vi "EZ Temperature.vi"(0 "VISA Resource Name":refnum<visa-resource-name>, 1 "Scan List (empty)":string, 5 "Thermocouple Type (8:Def-Last)":T2(ring)=enum."Default (Last)", 7 "Thermistor Type (3:Def-Last)":T3(ring)=enum."Default (Last)", 9 "RTD Type (2:Default-Last)":enum16{"85", "91", "Default (Last)"}(ring)=enum."Default (Last)", 11 "error in (no error)":errorcluster, 12 "Transducer Type (4:Def-Last)":T1(ring)=enum."Default (Last)") -> (4 "VISA Resource Name Out":refnum<visa-resource-name>, 8 "Output Array":dbl[](array[numeric]) format="%.2f", 15 "error out":errorcluster)   [LabVIEW 2016, in "Agilent 34970.lvlib"]
doc: "This VI lets you take simple temperature measurements. You can use various types of thermocouples, thermistors, or RTDs."
uses:
  Agilent 34970.lvlib
panel:
  out "concatenated string":string
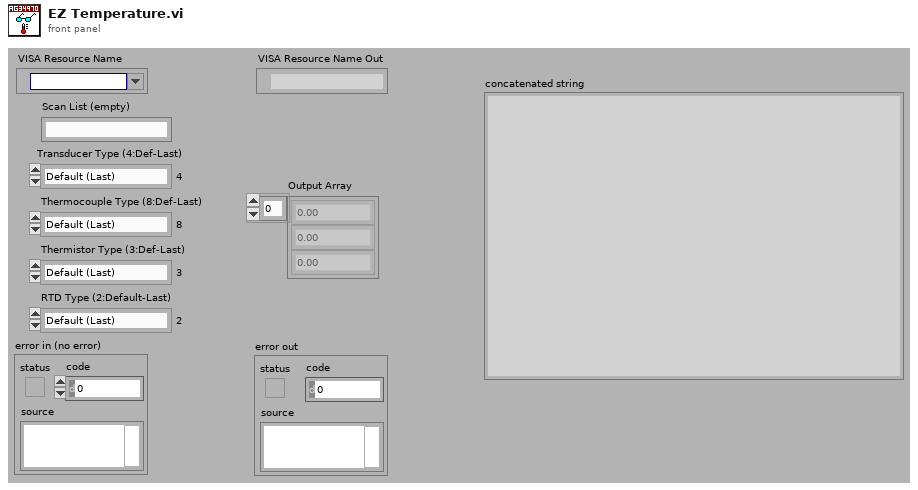
[diagram p1: front panel]
types:
  T1 = enum16{"Thermocouple", "Thermistor", "RTD", "4-Wire RTD", "Default (Last)"}
  T2 = enum16{"B", "E", "J", "K", "N", "R", "S", "T", "Default (Last)"}
  T3 = enum16{"2252", "5000", "10000", "Default (Last)"}
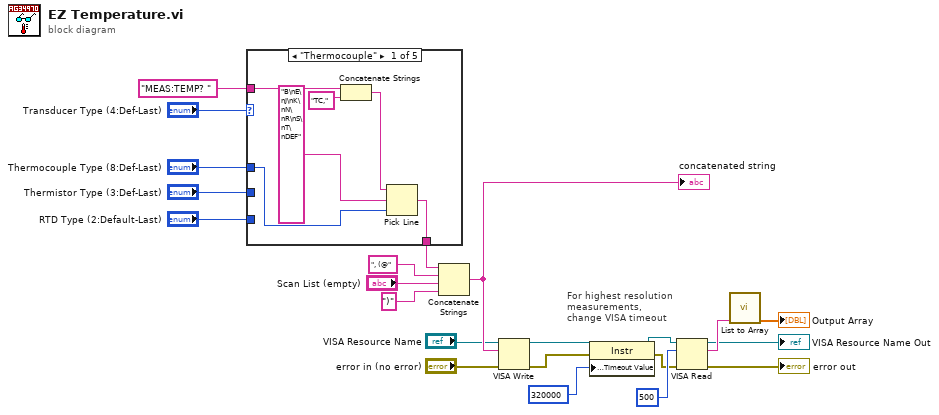
[diagram p0: block diagram]
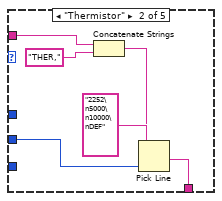
[diagram p2: hidden frame]
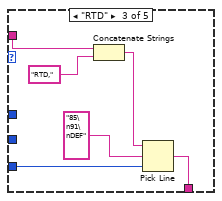
[diagram p3: hidden frame]
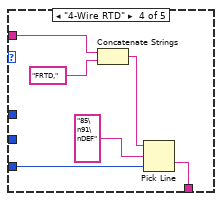
[diagram p4: hidden frame]
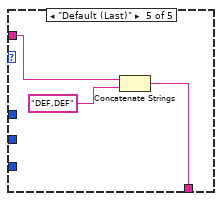
[diagram p5: hidden frame]
diagram:
  # "For highest resolution\nmeasurements, \nchange VISA timeout"
  n1 = case shown="\"Thermocouple\"" "Transducer Type (4:Def-Last)" {
    tunnel: "MEAS:TEMP? " -> [w27 w30 w37 w44 w48]
    tunnel: [w24 w31 w36 w45 w47] -> w12
    tunnel: "Thermocouple Type (8:Def-Last)" -> [w23 _ _ _ _]
    tunnel: "Thermistor Type (3:Def-Last)" -> [_ w29 _ _ _]
    tunnel: "RTD Type (2:Default-Last)" -> [_ _ w35 w43 _]
    frame "Thermocouple" {
      n2 = Concatenate Strings(w27, "TC,") -> (w25:string)
      n3 = Pick Line(string ("")=w25, multi-line string="B\nE\nJ\nK\nN\nR\nS\nT\nDEF", line index=w23) -> (output string=w24:string)
    }
    frame "Thermistor" {
      n4 = Concatenate Strings(w30, "THER,") -> (w32:string)
      n5 = Pick Line(string ("")=w32, multi-line string="2252\n5000\n10000\nDEF", line index=w29) -> (output string=w31:string)
    }
    frame "RTD" {
      n6 = Concatenate Strings(w37, "RTD,") -> (w40:string)
      n7 = Pick Line(string ("")=w40, multi-line string="85\n91\nDEF", line index=w35) -> (output string=w36:string)
    }
    frame "4-Wire RTD" {
      n8 = Concatenate Strings(w44, "FRTD,") -> (w41:string)
      n9 = Pick Line(string ("")=w41, multi-line string="85\n91\nDEF", line index=w43) -> (output string=w45:string)
    }
    frame "Default (Last)" {
      n10 = Concatenate Strings(w48, "DEF,DEF") -> (w47:string)
    }
  }
  n11 = Concatenate Strings(w12, ", (@", "Scan List (empty)", ")") -> (w11:string)
  "concatenated string" <- w11
  n12 = VISA Write(VISA resource name="VISA Resource Name", write buffer=w11, error in (no error)="error in (no error)") -> (VISA resource name out=w4:refnum<visa-resource-name>, error out=w3:errorcluster)  [unwired: 1 out]
  n13 = property class="Instr"(reference=w4, error in=w3, "General Settings:Timeout Value"=u32 320000 ("Tmo Value")) -> (reference out=w2:refnum<visa-resource-name>, error out=w1:errorcluster)
  n14 = VISA Read(VISA resource name=w2, byte count=u32 500 ("byte count (0)"), error in (no error)=w1) -> (VISA resource name out=→"VISA Resource Name Out":refnum<visa-resource-name>, read buffer=w13:string, error out=→"error out":errorcluster)  [unwired: 1 out]
  n15 = call "List to Array.vi"("List (empty)"=w13) -> ("Output Number Array"=→"Output Array":dbl[])  [unwired: 9 in, 1 out]
